vi "Write Write.vi"(8 "error in (no error)":errorcluster, 10 "Write":bool, 11 "myOtherClass in":refnum<class "myOtherClass.lvclass">) -> (0 "error out":errorcluster, 3 "myOtherClass out":refnum<class "myOtherClass.lvclass">)   [LabVIEW 2017, in "myOtherClass.lvclass"]
uses:
  myOtherClass.lvclass
  myOtherClass.lvclass/myOtherClass.ctl
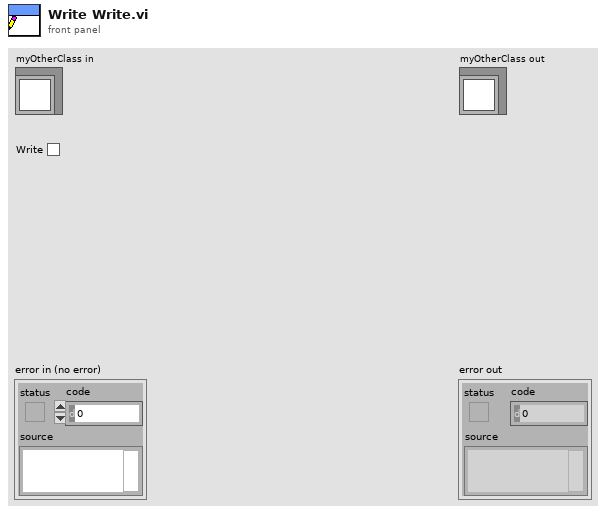
[diagram p1: front panel]
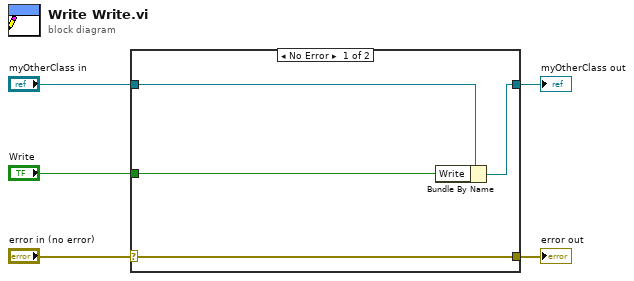
[diagram p0: block diagram]
diagram:
  n1 = case shown="No Error" "error in (no error)" {
    selector: "error in (no error)" -> [w9 w10]
    tunnel: [w9 w10] -> w4
    tunnel: [w7 w11] -> w2
    tunnel: "myOtherClass in" -> [w8 w11]
    tunnel: "Write" -> [w6 _]
    frame No Error {
      n2 = Bundle By Name(cluster=w8, "Write"=w6) -> (w7:refnum<class "myOtherClass.lvclass">)
    }
    frame Error {
    }
  }
  "error out" <- w4
  "myOtherClass out" <- w2
